vi "Configure the Buzzer.vi"(5 "Enable to Query":bool, 7 "Enable to Setup":bool, 8 "error in":errorcluster, 9 "Setup Buzzer Sound for FAIL":T3={"Buzzer Sound"=0, "Duration Time(Sec)"=0.2} {"Duration Time(Sec)" min=0.2 max=999.9 step=0.1 format="%#.1f"; "Buzzer Sound" format="%b" items=["ON"=1, "OFF"=0]}, 10 "Setup Buzzer Sound for PASS":T3={"Buzzer Sound"=0, "Duration Time(Sec)"=0.20000000298023224} {"Duration Time(Sec)" min=0.20000000298023224 max=999.9000244140625 step=0.1 format="%#.1f"; "Buzzer Sound" format="%b" items=["ON"=1, "OFF"=0]}, 11 "VISA resource name":refnum<visa-resource-name>) -> (0 "error out":errorcluster, 1 "Query Buzzer Sound for FAIL":T1, 2 "Query Buzzer Sound for PASS":T2, 3 "VISA resource name out":refnum<visa-resource-name>)   [LabVIEW 2011, in "GPT-9000.lvlib"]
uses:
  <instrlib>/GPT-9000/GPT-9000.lvlib
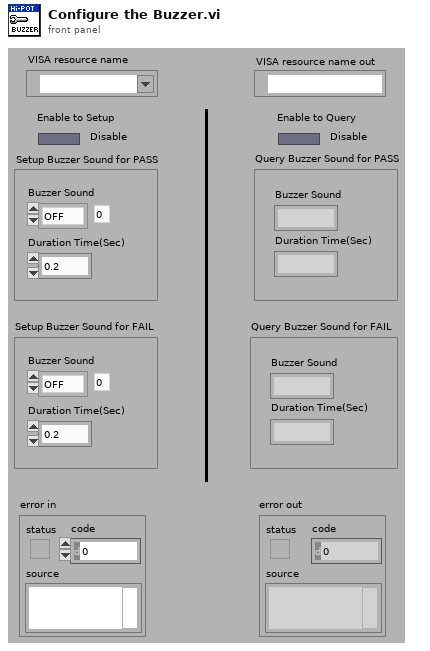
[diagram p1: front panel]
types:
  T1 = cluster{"Duration Time(Sec)":string, "Buzzer Sound":string}
  T2 = cluster{"Buzzer Sound":string, "Duration Time(Sec)":string}
  T3 = cluster{"Buzzer Sound":u8, "Duration Time(Sec)":dbl}
  T4 = cluster{"read buffer":string, "read buffer":string}
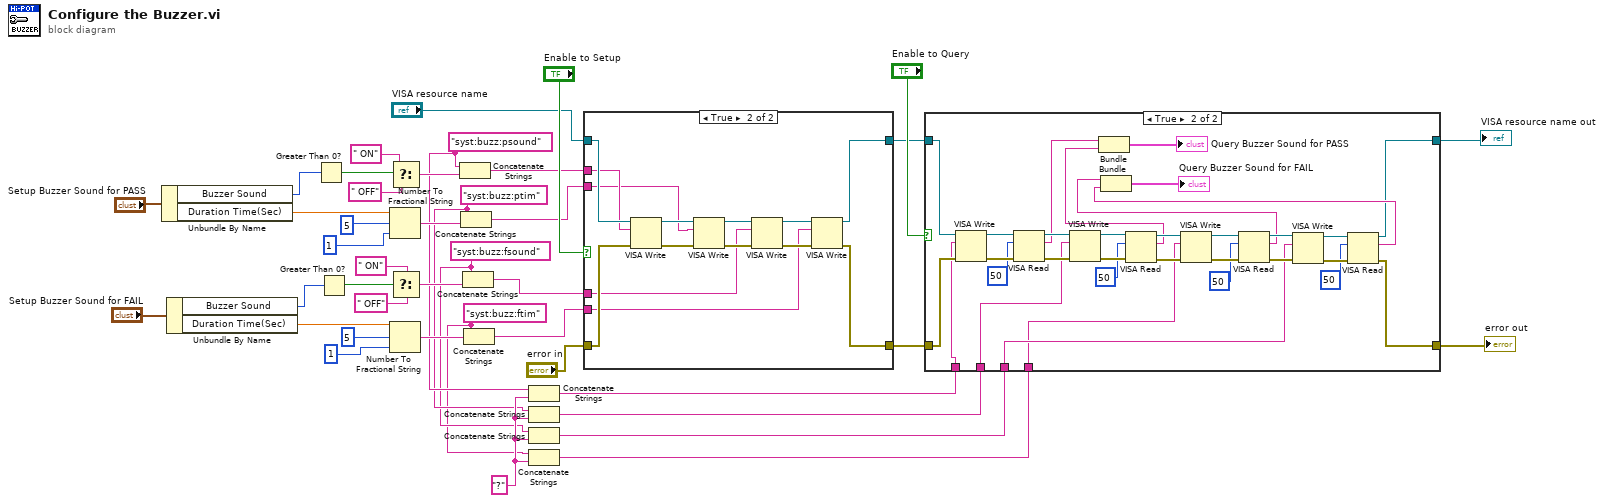
[diagram p0: block diagram]
diagram:
  w18 = "?" ("string")
  w14 = "syst:buzz:ftim" ("string")
  w15 = "syst:buzz:fsound" ("string")
  w16 = "syst:buzz:ptim" ("string")
  w17 = "syst:buzz:psound" ("string")
  n1 = Unbundle By Name("Setup Buzzer Sound for PASS") -> ("Buzzer Sound"=w4:u8, "Duration Time(Sec)"=w35:dbl)
  n2 = Unbundle By Name("Setup Buzzer Sound for FAIL") -> ("Buzzer Sound"=w1:u8, "Duration Time(Sec)"=w34:dbl)
  n3 = Greater Than 0?(x=w4) -> (x > 0?=w3:bool)
  n4 = Greater Than 0?(x=w1) -> (x > 0?=w2:bool)
  n5 = Number To Fractional String(number=w35, width (-)=i16 5, precision (6)=i16 1) -> (F-format string=w31:string)  [unwired: 1 in]
  n6 = Number To Fractional String(number=w34, width (-)=i16 5, precision (6)=i16 1) -> (F-format string=w29:string)  [unwired: 1 in]
  n7 = Select(t=" ON", s=w3, f=" OFF") -> (s? t:f=w32:string)
  n8 = Select(t=" ON", s=w2, f=" OFF") -> (s? t:f=w30:string)
  n9 = Concatenate Strings(w17, w32) -> (w27:string)
  n10 = Concatenate Strings(w16, w31) -> (w26:string)
  n11 = Concatenate Strings(w15, w30) -> (w25:string)
  n12 = Concatenate Strings(w14, w29) -> (w24:string)
  n13 = Concatenate Strings(w17, w18) -> (w13:string)
  n14 = Concatenate Strings(w16, w18) -> (w12:string)
  n15 = Concatenate Strings(w15, w18) -> (w11:string)
  n16 = Concatenate Strings(w14, w18) -> (w10:string)
  n17 = case shown="True" "Enable to Setup" {
    tunnel: w27 -> [_ w47]
    tunnel: w26 -> [_ w46]
    tunnel: w25 -> [_ w45]
    tunnel: w24 -> [_ w44]
    tunnel: "VISA resource name" -> [w43 w51]
    tunnel: "error in" -> [w42 w50]
    tunnel: [w43 w49] -> w9
    tunnel: [w42 w48] -> w8
    frame False {
    }
    frame True {
      n18 = VISA Write(VISA resource name=w51, write buffer=w47, error in (no error)=w50) -> (VISA resource name out=w56:refnum<visa-resource-name>, error out=w57:errorcluster)  [unwired: 1 out]
      n19 = VISA Write(VISA resource name=w56, write buffer=w46, error in (no error)=w57) -> (VISA resource name out=w54:refnum<visa-resource-name>, error out=w55:errorcluster)  [unwired: 1 out]
      n20 = VISA Write(VISA resource name=w54, write buffer=w45, error in (no error)=w55) -> (VISA resource name out=w52:refnum<visa-resource-name>, error out=w53:errorcluster)  [unwired: 1 out]
      n21 = VISA Write(VISA resource name=w52, write buffer=w44, error in (no error)=w53) -> (VISA resource name out=w49:refnum<visa-resource-name>, error out=w48:errorcluster)  [unwired: 1 out]
    }
  }
  n22 = case shown="True" "Enable to Query" {
    tunnel: w13 -> [_ w89]
    tunnel: w12 -> [_ w83]
    tunnel: w11 -> [_ w61]
    tunnel: w10 -> [_ w60]
    tunnel: w9 -> [w59 w91]
    tunnel: w8 -> [w58 w90]
    tunnel: [w59 w63] -> w7
    tunnel: [w58 w62] -> w6
    frame False {
    }
    frame True {
      n23 = VISA Write(VISA resource name=w91, write buffer=w89, error in (no error)=w90) -> (VISA resource name out=w87:refnum<visa-resource-name>, error out=w88:errorcluster)  [unwired: 1 out]
      n24 = VISA Read(VISA resource name=w87, byte count=u32 50, error in (no error)=w88) -> (VISA resource name out=w85:refnum<visa-resource-name>, read buffer=w69:string, error out=w84:errorcluster)  [unwired: 1 out]
      n25 = VISA Write(VISA resource name=w85, write buffer=w83, error in (no error)=w84) -> (VISA resource name out=w81:refnum<visa-resource-name>, error out=w82:errorcluster)  [unwired: 1 out]
      n26 = VISA Read(VISA resource name=w81, byte count=u32 50, error in (no error)=w82) -> (VISA resource name out=w78:refnum<visa-resource-name>, read buffer=w68:string, error out=w79:errorcluster)  [unwired: 1 out]
      n27 = Bundle("read buffer"=w69, "read buffer"=w68) -> (→"Query Buzzer Sound for PASS":T4)  [unwired: 1 in]
      n28 = VISA Write(VISA resource name=w78, write buffer=w60, error in (no error)=w79) -> (VISA resource name out=w77:refnum<visa-resource-name>, error out=w76:errorcluster)  [unwired: 1 out]
      n29 = VISA Read(VISA resource name=w77, byte count=u32 50, error in (no error)=w76) -> (VISA resource name out=w74:refnum<visa-resource-name>, read buffer=w66:string, error out=w73:errorcluster)  [unwired: 1 out]
      n30 = VISA Write(VISA resource name=w74, write buffer=w61, error in (no error)=w73) -> (VISA resource name out=w71:refnum<visa-resource-name>, error out=w72:errorcluster)  [unwired: 1 out]
      n31 = VISA Read(VISA resource name=w71, byte count=u32 50, error in (no error)=w72) -> (VISA resource name out=w63:refnum<visa-resource-name>, read buffer=w65:string, error out=w62:errorcluster)  [unwired: 1 out]
      n32 = Bundle("read buffer"=w66, "read buffer"=w65) -> (→"Query Buzzer Sound for FAIL":T4)  [unwired: 1 in]
    }
  }
  "VISA resource name out" <- w7
  "error out" <- w6
